vi "Mouse Control.vi"() -> ()   [LabVIEW 2021]
uses:
  <vilib>/Utility/inputDevices.llb/mouseAcquire.vi
  <vilib>/Utility/inputDevices.llb/closeMouse.vi
panel:
  out "Vertical":i32
  out "Horizontal":i32
  out "Right Click":bool
  out "Left Click":bool
  in  "stop":bool
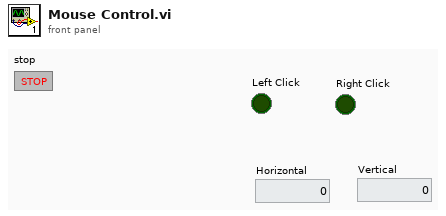
[diagram p1: front panel]
types:
  T1 = cluster{"Horizontal":i32, "Vertical":i32, "Scrolling":i32}
  T2 = cluster{"button 1":bool, "button 2":bool, "button 3":bool, "button 4":bool}
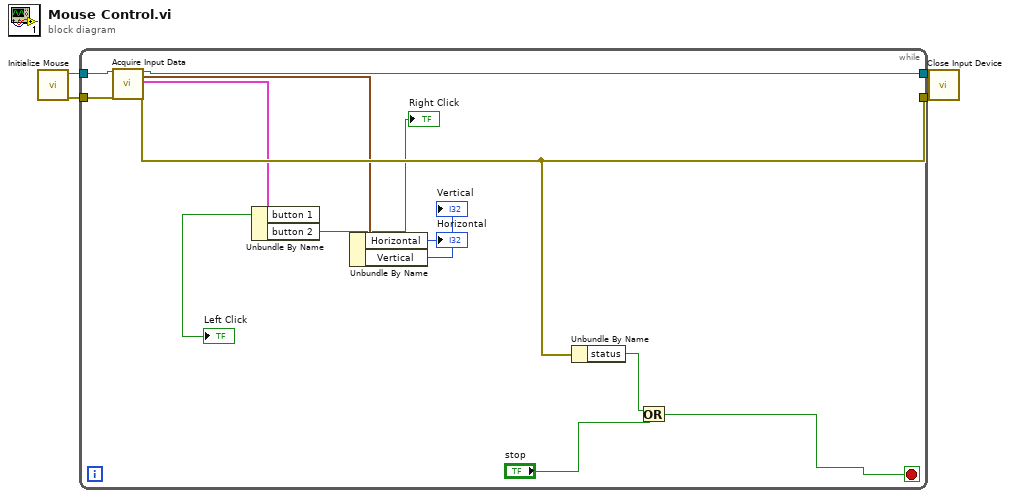
[diagram p0: block diagram]
diagram:
  n1 = call <vilib>:"Initialize Mouse.vi"() -> ("error out"=w1:errorcluster, "device ID"=w2:refnum<k1>)  [unwired: 10 in]
  n2 = while {
    tunnel: [w17] -> w4
    tunnel: [w14] -> w3
    tunnel: w2 -> [w16]
    tunnel: w1 -> [w15]
    stop <- w12 stop-if-true
    n3 = call-poly <vilib>:"Acquire Input Data.vi"("device ID"=w16, "error in (no error)"=w15) -> ("device ID"=w17:refnum<k1>, "axis info"=w11:T1, "button info"=w10:T2, "error out"=w14:errorcluster)  [unwired: 14 in]
    n4 = Unbundle By Name(w10) -> ("button 1"=→"Left Click":bool, "button 2"=→"Right Click":bool)
    n5 = Unbundle By Name(w11) -> ("Horizontal"=→"Horizontal":i32, "Vertical"=→"Vertical":i32)
    n6 = Unbundle By Name(w14) -> ("status"=w13:bool)
    n7 = Or(x=w13, y="stop") -> (x .or. y?=w12:bool)
  }
  n8 = call-poly <vilib>:"Close Input Device.vi"("error in (no error)"=w3, "device ID"=w4) -> ()  [unwired: 8 in, 1 out]
